vi "Create.vi"(8 "error in (no error)":errorcluster, 11 "SSE Ref":refnum<data-value>) -> (0 "error out":errorcluster, 3 "SSE Handler out":refnum<class "SSE Handler.lvclass">)   [LabVIEW 2020, in "HTTP Server.lvlib" / "SSE Handler.lvclass"]
uses:
  SSE Handler.lvclass
  SSE Handler.lvclass/SSE Handler.ctl
  SSE Manager/SSE Manager.lvclass
  Server Sent Events Data.ctl
  HTTP Server.lvlib
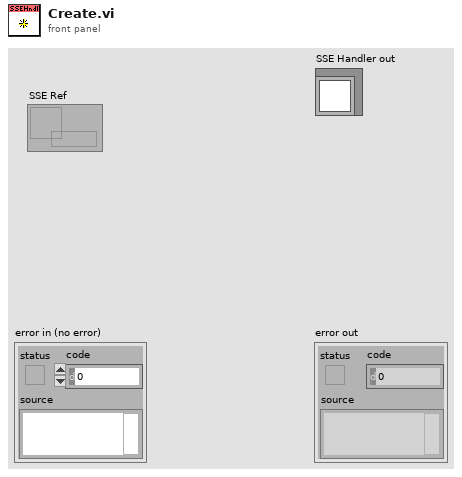
[diagram p1: front panel]
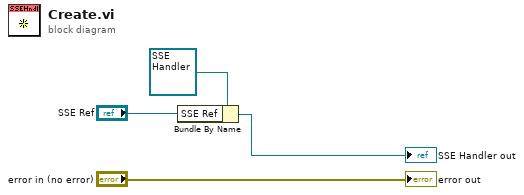
[diagram p0: block diagram]
diagram:
  n1 = Bundle By Name(cluster=refnum<class "SSE Handler.lvclass"> refnum ("SSE Handler in"), "SSE Ref"="SSE Ref") -> (→"SSE Handler out":refnum<class "SSE Handler.lvclass">)
  "error out" <- "error in (no error)"
